vi "area.vi"(11 "radius":dbl) -> (3 "function return":dbl)   [LabVIEW 2013, in "CircularArea.lvlib"]
doc: "__declspec(dllexport) double area(double radius);"
uses:
  CircularArea.lvlib
  CircularArea.dll
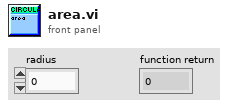
[diagram p1: front panel]
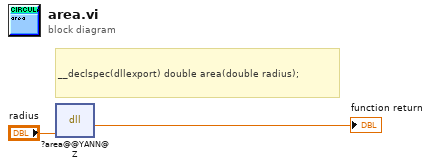
[diagram p0: block diagram]
diagram:
  # "__declspec(dllexport) double area(double radius);"
  n1 = dll-call lib="D:/congxin/labview/CircularArea.*" fn="?area@@YANN@Z"("radius"="radius") -> (→"function return":dbl)  [unwired: 4 in, 2 out]
